vi "Check_with_Jump_PN.vi"(0 "Current position":sgl[](array[numeric])=[0.0, 200.0, 40.0] format="%.2f", 1 "Traverse Name":string, 3 "Simulate/Run":T1=enum."Run VI", 5 "New Position":sgl[](array[numeric])=[0.0, 100.0, 40.0] format="%.2f", 7 "Traverse Active Parts":cluster{"X":bool, "XY":bool, "XYZ":bool}, 14 "Model       Roll      Pitch       Yaw (deg)":sgl[](array[numeric]) format="%#.2f") -> (4 "Error Comments":string, 10 "Steps":sgl[][](array[numeric])=[[0.0, 200.0, 40.0]] format="%.2f")   [LabVIEW 2022 SP3]
uses:
  Controls/User_Specific_mode.ctl
  Collision_Detection/Triangles/EnFlo specific/Collision Mode.ctl
  Route_mapping_global.vi
  Globals/Trav_pos_global.vi
  Globals/Constants_global.vi
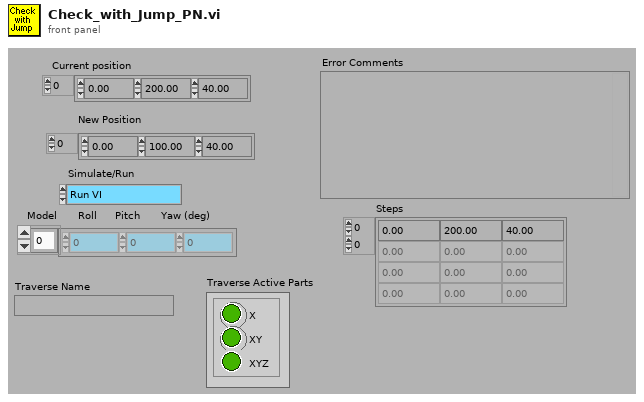
[diagram p1: front panel]
types:
  T1 = typedef "User_Specific_mode.ctl" = enum16{"Check VI only", "Run VI"}
  T2 = typedef "Box_size.ctl" = cluster{"Max":sgl, "Min":sgl}[]
  T3 = typedef "Collision Mode.ctl" = enum16{"Traverse - Tunnel", "Traverse - Model", "Traverse - Fixed objects", "Traverse - Traverse", "Traverse - All"}
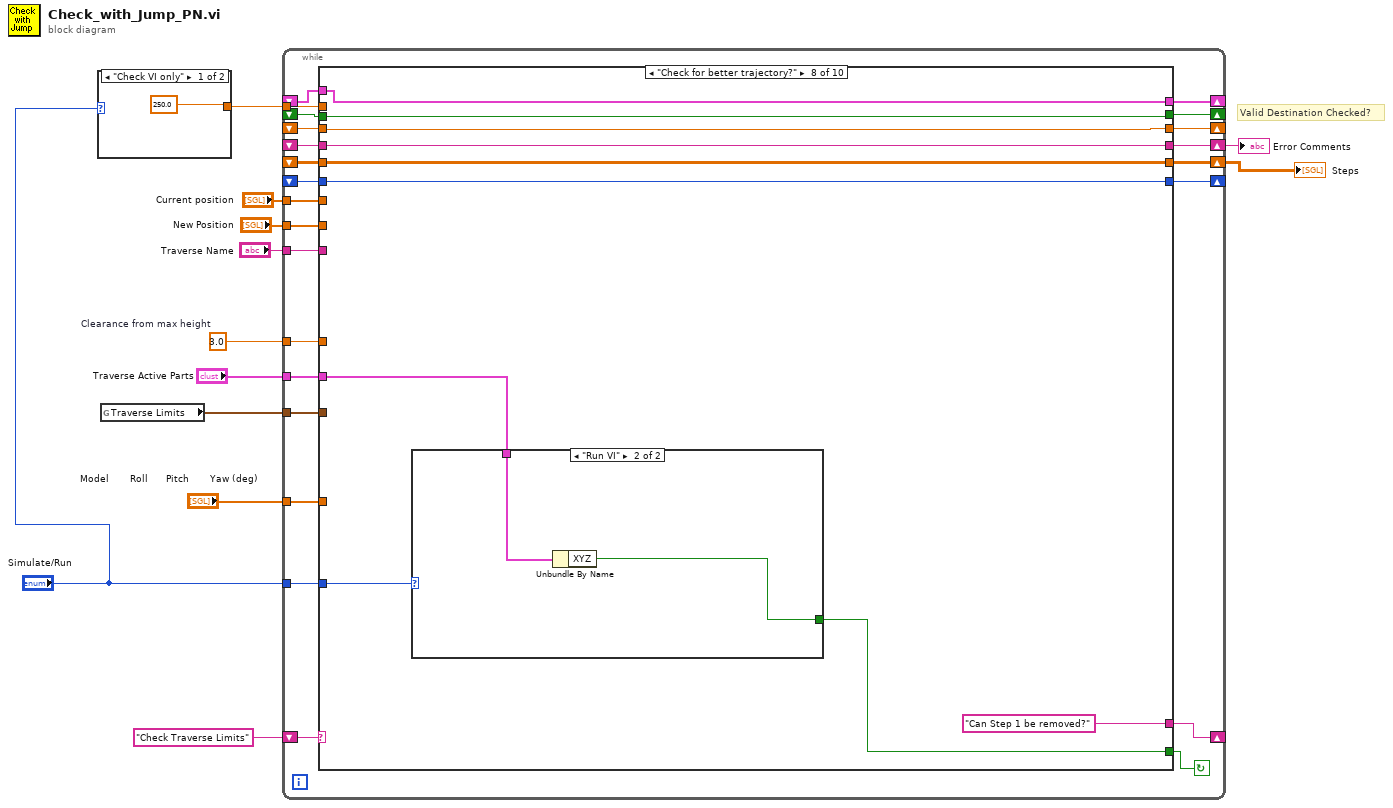
[diagram p0: block diagram]
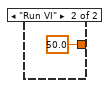
[diagram p2: hidden frame]
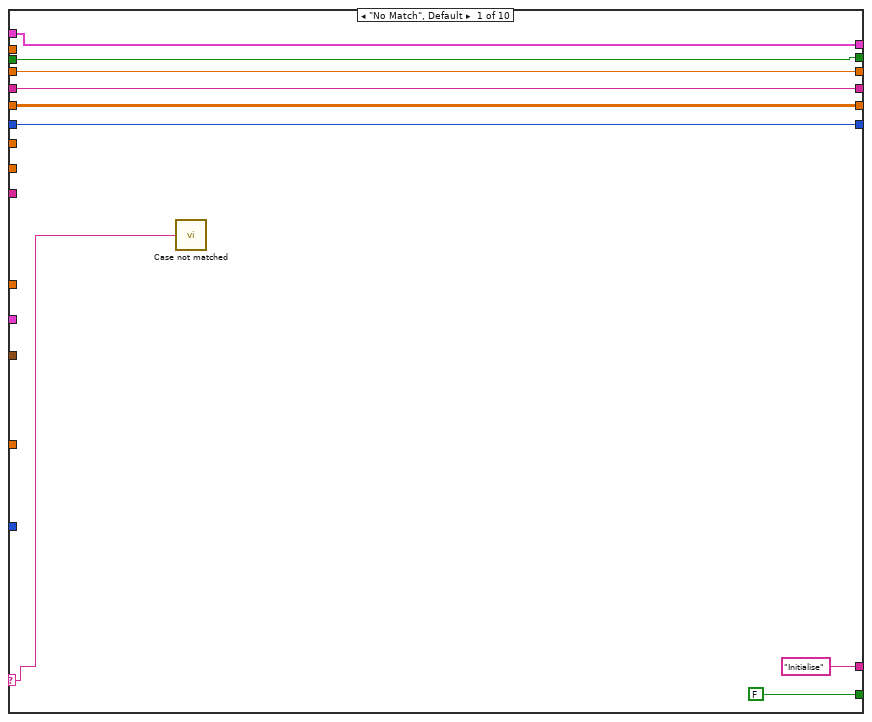
[diagram p3: hidden frame]
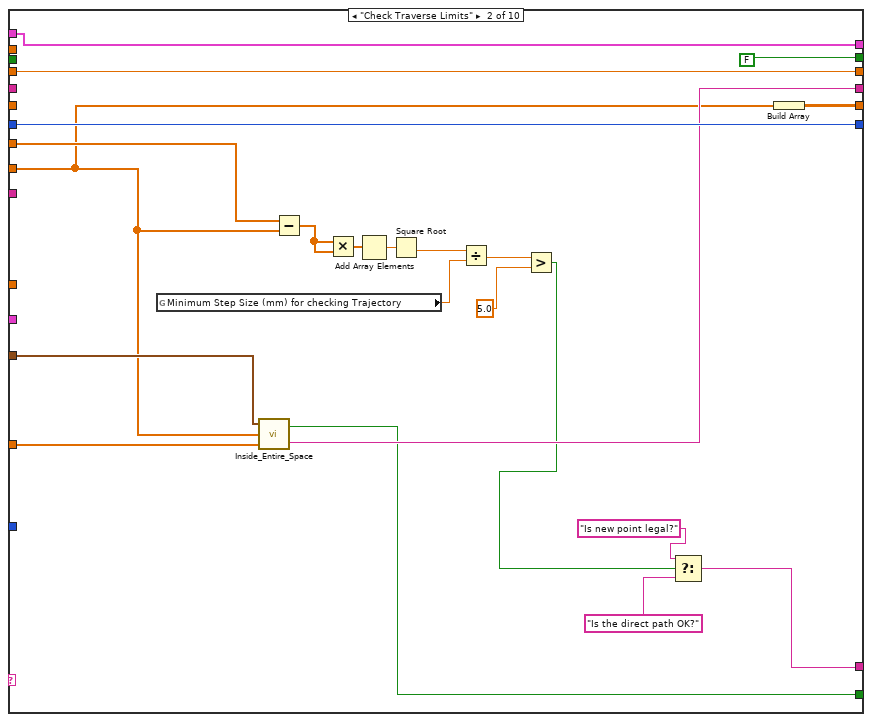
[diagram p4: hidden frame]
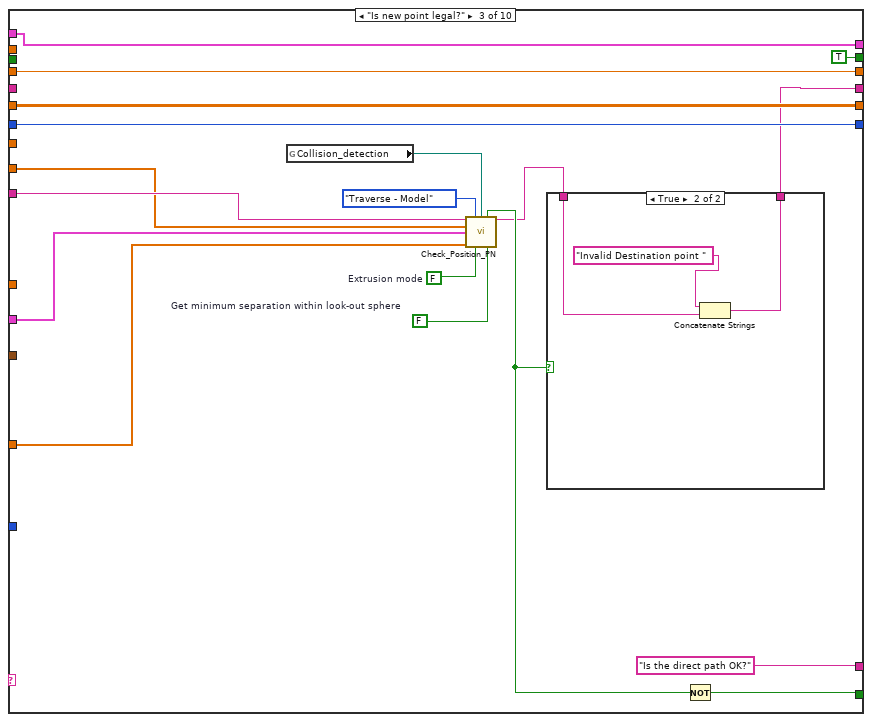
[diagram p5: hidden frame]
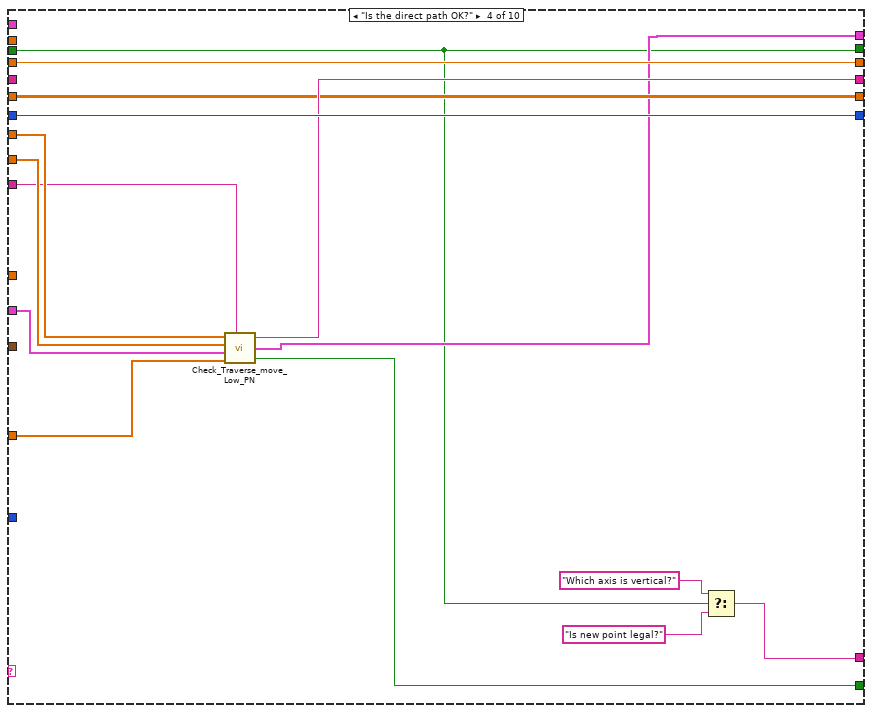
[diagram p7: hidden frame]
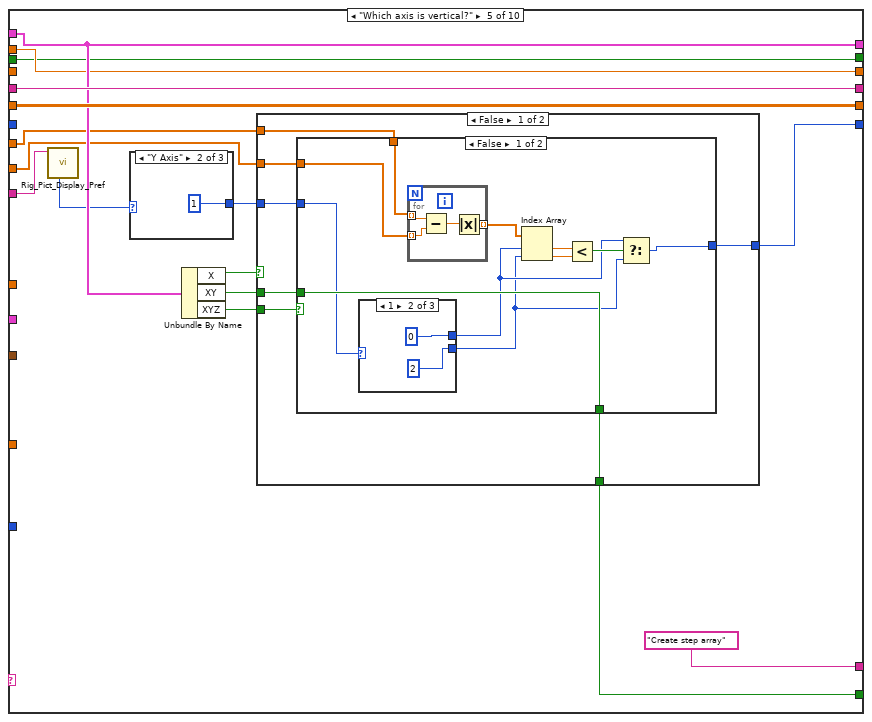
[diagram p8: hidden frame]
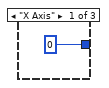
[diagram p9: hidden frame]
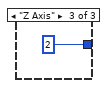
[diagram p10: hidden frame]
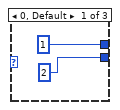
[diagram p11: hidden frame]
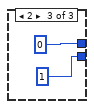
[diagram p12: hidden frame]
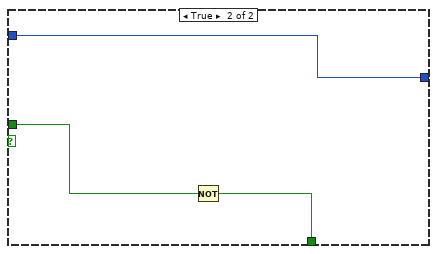
[diagram p13: hidden frame]
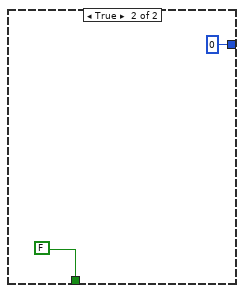
[diagram p14: hidden frame]
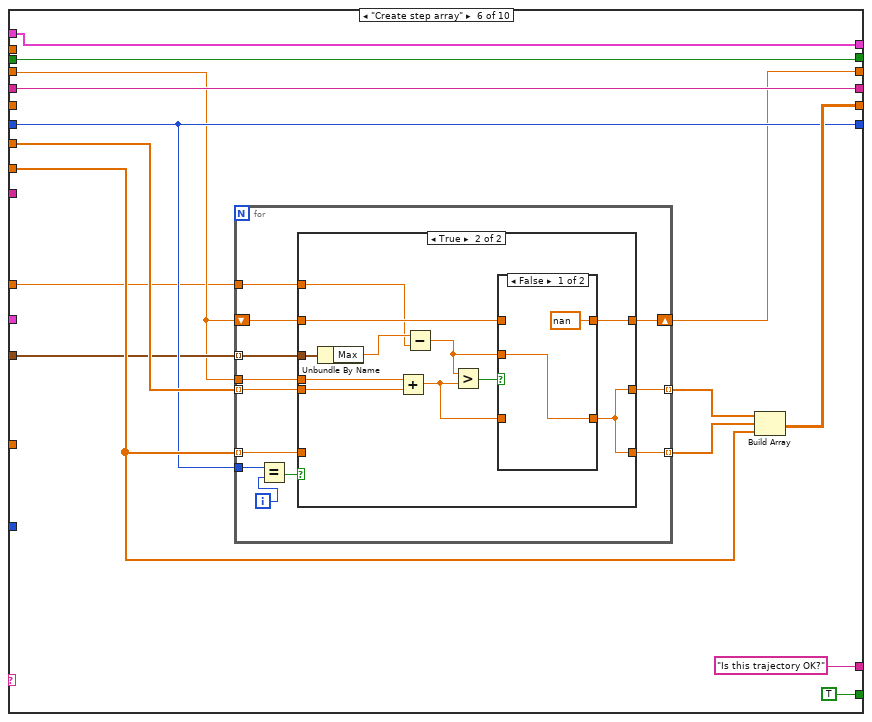
[diagram p15: hidden frame]
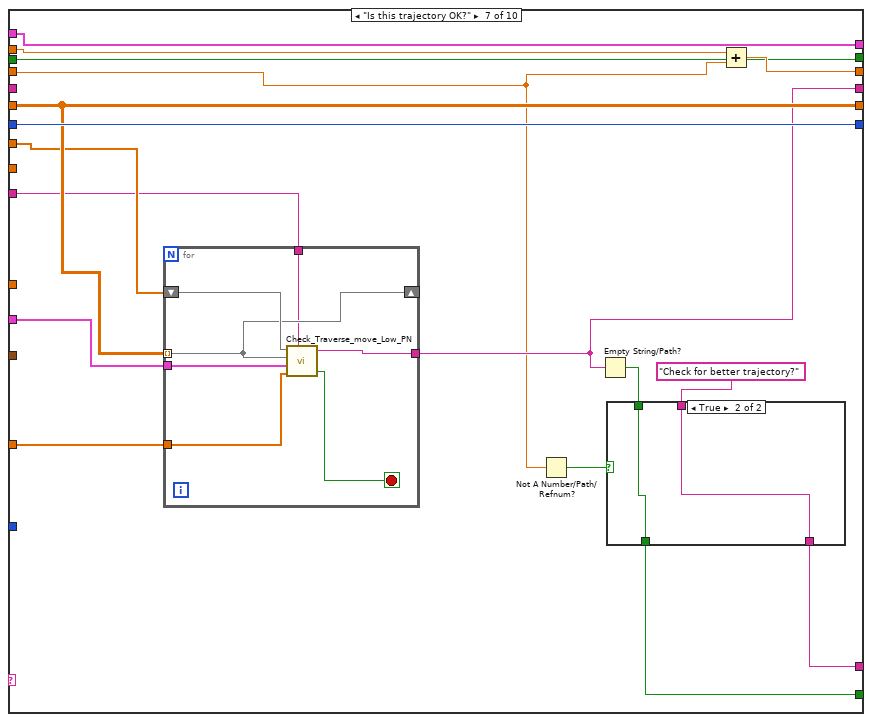
[diagram p18: hidden frame]
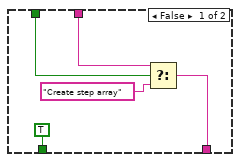
[diagram p19: hidden frame]
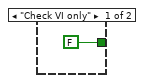
[diagram p20: hidden frame]
diagram:
  w3 = sgl 3.0  # Clearance from max height
  # "Valid Destination Checked?"
  n1 = case shown="\"Check VI only\"" "Simulate/Run" {
    tunnel: [sgl 250.0 sgl 50.0] -> w10
    frame "Check VI only" {
    }
    frame "Run VI" {
    }
  }
  n2 = global read "Route_mapping_global.vi" "Traverse Limits"() -> (w4:T2)
  n3 = while {
    shift-left: "Check Traverse Limits" -> [w22]
    shift-right: [w38] -> _
    shift-right: [w35] -> w8
    shift-left: _ -> [w36]
    shift-right: [w34] -> w7
    shift-left: _ -> [w33]
    tunnel: "Current position" -> [w32]
    tunnel: "New Position" -> [w31]
    tunnel: "Traverse Name" -> [w30]
    shift-right: [w29] -> _
    shift-left: _ -> [w28]
    shift-right: [w27] -> _
    shift-left: _ -> [w26]
    tunnel: w10 -> [w25]
    tunnel: "Simulate/Run" -> [w24]
    tunnel: "Model       Roll      Pitch       Yaw (deg)" -> [w23]
    tunnel: w4 -> [w21]
    tunnel: w3 -> [w20]
    shift-right: [w19] -> _
    shift-left: _ -> [w18]
    tunnel: "Traverse Active Parts" -> [w17]
    shift-right: [w16] -> _
    shift-left: _ -> [w15]
    stop <- w37 continue-if-true
    n4 = case shown="\"Check for better trajectory?\"" w22 {
      selector: w22 -> [w39 _ _ _ _ _ _ _ _ _]
      tunnel: [FALSE w63 w77 w99 w116 TRUE w208 w238 w251 FALSE] -> w37
      tunnel: ["Initialise" w49 "Is the direct path OK?" w92 "Create step array" "Is this trajectory OK?" w218 "Can Step 1 be removed?" w256 "End"] -> w38
      tunnel: w36 -> [w45 _ _ _ w120 w172 _ w244 _ _]
      tunnel: [w45 w64 w72 w100 w120 w172 w209 w244 "" ""] -> w35
      tunnel: [w44 w67 w84 w98 w121 w166 w213 w241 w260 w286] -> w34
      tunnel: w33 -> [w44 _ w84 w98 w121 _ w213 w241 w259 w281]
      tunnel: w32 -> [_ w61 _ w104 w109 w170 w212 _ w255 _]
      tunnel: w31 -> [_ w60 w79 w103 w108 w167 _ _ _ _]
      tunnel: w30 -> [_ _ w80 w101 w111 _ w210 _ w252 w277]
      tunnel: [w43 w68 w86 w105 w119 w165 w220 w243 w262 w288] -> w29
      tunnel: w28 -> [w43 w68 w86 w105 _ w165 w220 w243 w262 w288]
      tunnel: [w42 w69 w87 w106 w113 w162 w216 w242 w258 w285] -> w27
      tunnel: w26 -> [w42 w69 w87 w106 _ w163 w205 w242 w258 w285]
      tunnel: w25 -> [_ _ _ _ w113 _ w217 _ _ _]
      tunnel: w24 -> [_ _ _ _ _ _ _ w240 _ _]
      tunnel: w23 -> [_ w65 w78 w102 _ _ w211 _ w253 w278]
      tunnel: w21 -> [_ w66 _ _ _ w164 _ _ _ _]
      tunnel: w20 -> [_ _ _ _ _ w161 _ _ _ _]
      tunnel: [w41 w62 w76 w97 w118 w160 w207 w237 w250 w274] -> w19
      tunnel: w18 -> [w41 w62 w76 _ w118 w160 w207 w237 w250 w274]
      tunnel: w17 -> [_ _ w75 w96 _ _ w206 w236 w249 w273]
      tunnel: [w40 FALSE TRUE w95 w107 w159 w204 w235 w248 w272] -> w16
      tunnel: w15 -> [w40 _ _ w95 w107 w159 w204 w235 w248 w272]
      frame "No Match", Default {
        n5 = call "Case not matched.vi"("Case Name not Matched"=w39) -> ()
      }
      frame "Check Traverse Limits" {
        n6 = global read "Trav_pos_global.vi" "Minimum Step Size (mm) for checking Trajectory"() -> (w55:sgl)
        n7 = call "Inside_Entire_Space.vi"("Model       Roll      Pitch       Yaw (deg)"=w65, "Current Position"=w60, "Envelope"=w66) -> ("Error Comments"=w64:string, "Box Inside"=w63:bool)  [unwired: 1 in]
        n8 = Subtract(x=w61, y=w60) -> (x-y=w59:sgl[])
        n9 = Multiply(x=w59, y=w59) -> (x*y=w58:sgl[])
        n10 = Add Array Elements(numeric array=w58) -> (sum=w57:sgl)
        n11 = Square Root(x=w57) -> (sqrt(x)=w56:sgl)
        n12 = Divide(x=w56, y=w55) -> (x/y=w54:sgl)
        n13 = Greater?(x=w54, y=sgl 5.0) -> (0:w52:bool)
        n14 = Select(t="Is new point legal?", s=w52, f="Is the direct path OK?") -> (s? t:f=w49:string)
        n15 = Build Array(w60) -> (w67:sgl[][])
      }
      frame "Is new point legal?" {
        w83 = FALSE  # Get minimum separation within look-out sphere
        w82 = FALSE  # Extrusion mode
        n16 = global read "Constants_global.vi" "Collision_detection"() -> (w70:path)
        n17 = call "Check_Position_PN.vi"("Traverse Name"=w80, "Collision mode"=Collision_Mode."Traverse - Model", "Collision_detection"=w70, "Position to check"=w79, "Traverse Active Parts"=w75, "Model Rotation (deg)"=w78, "Extrusion mode"=w82, "Get minimum separation within look-out sphere"=w83) -> ("Collision"=w74:bool, "Error Comments"=w73:string)  [unwired: 3 in, 3 out]
        n18 = case shown="True" w74 {
          tunnel: w73 -> [w88 w90]
          tunnel: [w88 w89] -> w72
          frame False {
          }
          frame True {
            n19 = Concatenate Strings("Invalid Destination point ", w90) -> (w89:string)
          }
        }
        n20 = Not(x=w74) -> (.not. x?=w77:bool)
      }
      frame "Is the direct path OK?" {
        n21 = call "Check_Traverse_move_Low_PN.vi"("Current position"=w104, "New Position"=w103, "Traverse Active Parts"=w96, "Model       Roll      Pitch       Yaw (deg)"=w102, "Traverse Name"=w101) -> ("Error Comments"=w100:string, "Traverse collision part"=w97:cluster{"X":bool, "XY":bool, "XYZ":bool}, "Collision"=w99:bool)
        n22 = Select(t="Which axis is vertical?", s=w95, f="Is new point legal?") -> (s? t:f=w92:string)
      }
      frame "Which axis is vertical?" {
        n23 = call "Rig_Pict_Display_Pref.vi"("Traverse Name"=w111) -> ("Which Axis is vertical?"=w112:enum16{"X Axis", "Y Axis", "Z Axis"})  [unwired: 7 out]
        n24 = case shown="\"Y Axis\"" w112 {
          tunnel: [0 1 2] -> w110
          frame "X Axis" {
          }
          frame "Y Axis" {
          }
          frame "Z Axis" {
          }
        }
        n25 = Unbundle By Name(w118) -> ("X"=w117:bool, "XY"=w114:bool, "XYZ"=w115:bool)
        n26 = case shown="False" w117 {
          tunnel: [w132 0] -> w119
          tunnel: [w129 FALSE] -> w116
          tunnel: w115 -> [w131 _]
          tunnel: w114 -> [w130 _]
          tunnel: w110 -> [w128 _]
          tunnel: w109 -> [w127 _]
          tunnel: w108 -> [w126 _]
          frame False {
            n27 = case shown="False" w131 {
              tunnel: [w133 w154] -> w132
              tunnel: w130 -> [w143 w156]
              tunnel: [w143 w155] -> w129
              tunnel: w128 -> [w142 w154]
              tunnel: w127 -> [w141 _]
              tunnel: w126 -> [w140 _]
              frame False {
                n28 = case shown="1" w142 {
                  tunnel: [1 0 0] -> w135
                  tunnel: [2 2 1] -> w134
                  frame 0, Default {
                  }
                  frame 1 {
                  }
                  frame 2 {
                  }
                }
                n29 = for {
                  tunnel: w141 -> [w147] mode=indexing
                  tunnel: w140 -> [w146] mode=indexing
                  tunnel: [w144] -> w139 mode=indexing
                  n30 = Subtract(x=w147, y=w146) -> (x-y=w145:sgl)
                  n31 = Absolute Value(x=w145) -> (abs(x)=w144:sgl)
                }
                n32 = Index Array(array=w139, index #1=w135, index #2=w134) -> (element #1=w137:sgl, element #2=w138:sgl)
                n33 = Less?(x=w137, y=w138) -> (x < y?=w136:bool)
                n34 = Select(t=w135, s=w136, f=w134) -> (s? t:f=w133:i32)
              }
              frame True {
                n35 = Not(x=w156) -> (.not. x?=w155:bool)
              }
            }
          }
          frame True {
          }
        }
      }
      frame "Create step array" {
        n36 = for {
          tunnel: w163 -> [w185]
          tunnel: w165 -> [w182]
          tunnel: w170 -> [w181] mode=indexing
          tunnel: [w180] -> w169 mode=indexing
          tunnel: w167 -> [w179] mode=indexing
          tunnel: [w178] -> w168 mode=indexing
          tunnel: w164 -> [w177] mode=indexing
          shift-right: [w175] -> w162
          shift-left: w163 -> [w176]
          tunnel: w161 -> [w174]
          i -> [w184]
          n37 = Equal?(x=w182, y=w184) -> (x = y?=w183:bool)
          n38 = case shown="True" w183 {
            tunnel: w185 -> [_ w199]
            tunnel: w181 -> [w188 w198]
            tunnel: [w188 w195] -> w180
            tunnel: w179 -> [w187 _]
            tunnel: [w187 w195] -> w178
            tunnel: w177 -> [_ w197]
            tunnel: w176 -> [w186 w192]
            tunnel: [w186 w193] -> w175
            tunnel: w174 -> [_ w189]
            frame False {
            }
            frame True {
              n39 = Unbundle By Name(w197) -> ("Max"=w191:sgl)
              n40 = Add(x=w199, y=w198) -> (x+y=w194:sgl)
              n41 = Subtract(x=w191, y=w189) -> (x-y=w190:sgl)
              n42 = Greater?(x=w190, y=w194) -> (0:w196:bool)
              n43 = case shown="False" w196 {
                tunnel: [w200 w203] -> w195
                tunnel: w194 -> [_ w203]
                tunnel: [sgl nan w202] -> w193
                tunnel: w192 -> [_ w202]
                tunnel: w190 -> [w200 _]
                frame False {
                }
                frame True {
                }
              }
            }
          }
        }
        n44 = Build Array(w169, w168, w167) -> (w166:sgl[][])
      }
      frame "Is this trajectory OK?" {
        n45 = for {
          tunnel: w213 -> [w226] mode=indexing
          shift-right: [w226] -> _
          shift-left: w212 -> [w227]
          tunnel: w211 -> [w225]
          tunnel: w210 -> [w224]
          tunnel: [w222] -> w209
          tunnel: w206 -> [w221]
          stop <- w223 stop-if-true
          n46 = call "Check_Traverse_move_Low_PN.vi"("Current position"=w227, "New Position"=w226, "Traverse Active Parts"=w221, "Model       Roll      Pitch       Yaw (deg)"=w225, "Traverse Name"=w224) -> ("Error Comments"=w222:string, "Collision"=w223:bool)  [unwired: 1 out]
        }
        n47 = Not A Number/Path/Refnum?(number/path/refnum=w205) -> (NaN/Path/Refnum?=w215:bool)
        n48 = Empty String/Path?(string/path=w209) -> (empty?=w219:bool)
        n49 = case shown="True" w215 {
          tunnel: w219 -> [w232 w233]
          tunnel: [w231 w234] -> w218
          tunnel: "Check for better trajectory?" -> [w229 w234]
          tunnel: [TRUE w233] -> w208
          frame False {
            n50 = Select(t=w229, s=w232, f="Create step array") -> (s? t:f=w231:string)
          }
          frame True {
          }
        }
        n51 = Add(x=w217, y=w205) -> (x+y=w216:sgl)
      }
      frame "Check for better trajectory?" {
        n52 = case shown="\"Run VI\"" w240 {
          tunnel: [FALSE w246] -> w238
          tunnel: w236 -> [_ w247]
          frame "Check VI only" {
          }
          frame "Run VI" {
            n53 = Unbundle By Name(w247) -> ("XYZ"=w246:bool)
          }
        }
      }
      frame "Can Step 1 be removed?" {
        n54 = Index Array(array=w259, index (row)=1) -> (element=w254:sgl[])  [unwired: 1 in]
        n55 = call "Check_Traverse_move_Low_PN.vi"("Current position"=w255, "New Position"=w254, "Traverse Active Parts"=w249, "Model       Roll      Pitch       Yaw (deg)"=w253, "Traverse Name"=w252) -> ("Collision"=w251:bool)  [unwired: 2 out]
        n56 = case shown="True" w251 {
          tunnel: [w264 w271] -> w260
          tunnel: w259 -> [w267 w271]
          tunnel: ["End" "Can Step 2 be removed?"] -> w256
          frame False {
            n57 = Index Array(array=w267, index (row)=1) -> (element=w266:sgl[])  [unwired: 1 in]
            n58 = Index Array(array=w267, index (row)=2) -> (element=w265:sgl[])  [unwired: 1 in]
            n59 = Build Array(w266, w265) -> (w264:sgl[][])
          }
          frame True {
          }
        }
      }
      frame "Can Step 2 be removed?" {
        n60 = Index Array(array=w281, index (row)=2) -> (element=w279:sgl[])  [unwired: 1 in]
        n61 = Index Array(array=w281, index (row)=0) -> (element=w280:sgl[])  [unwired: 1 in]
        n62 = call "Check_Traverse_move_Low_PN.vi"("Current position"=w280, "New Position"=w279, "Traverse Active Parts"=w273, "Model       Roll      Pitch       Yaw (deg)"=w278, "Traverse Name"=w277) -> ("Collision"=w276:bool)  [unwired: 2 out]
        n63 = case shown="False" w276 {
          tunnel: [w289 w295] -> w286
          tunnel: w281 -> [w292 w295]
          frame False {
            n64 = Index Array(array=w292, index (row)=0) -> (element=w291:sgl[])  [unwired: 1 in]
            n65 = Index Array(array=w292, index (row)=2) -> (element=w290:sgl[])  [unwired: 1 in]
            n66 = Build Array(w291, w290) -> (w289:sgl[][])
          }
          frame True {
          }
        }
      }
    }
  }
  "Error Comments" <- w8
  "Steps" <- w7
